vi "Clear.vi"(8 "Error In":errorcluster, 11 "Tree Control In":refnum<vi>) -> (0 "Error Out":errorcluster, 3 "Tree Control Out":refnum<vi>)   [LabVIEW 2018, in "TraceTreeEditor.lvlib"]
uses:
  TraceTreeEditor.lvlib
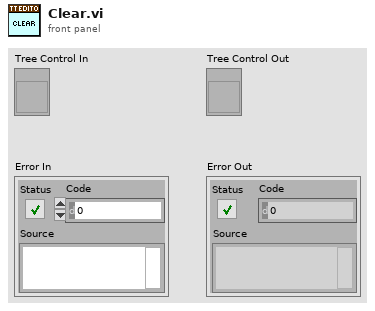
[diagram p1: front panel]
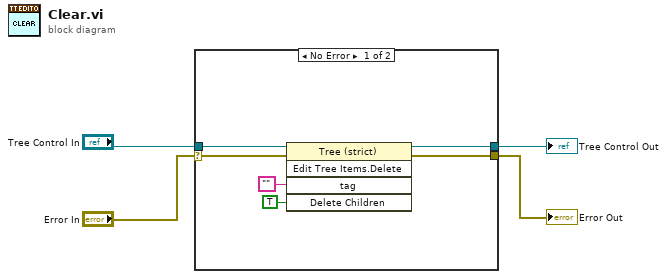
[diagram p0: block diagram]
diagram:
  n1 = case shown="No Error" "Error In" {
    selector: "Error In" -> [w10 w12]
    tunnel: [w8 w11] -> w2
    tunnel: "Tree Control In" -> [w7 w11]
    tunnel: [w9 w12] -> w3
    frame No Error {
      n2 = invoke class="Tree (strict)" method="Edit Tree Items.Delete"(reference=w7, error in=w10, "tag"="", "Delete Children"=TRUE ("Delete Children?")) -> (reference out=w8:refnum<vi>, error out=w9:errorcluster)  [unwired: 1 in, 3 out]
    }
    frame Error {
    }
  }
  "Tree Control Out" <- w2
  "Error Out" <- w3
